vi "GE 5565PIORC.DMA.Scatter-Gather.Link Block Descriptors.vi"(8 "error in (no error)":errorcluster, 10 "Block Descriptors":T1[](array[typedef]) {"descriptor params"."data ptr (lower)" format="%.0x"; "descriptor params"."data ptr (upper)" format="%.0x"; "descriptor params"."data size" format="%.0x"; "descriptor params"."next descriptor ptr" format="%.0x"; "descriptor size" format="%08x"; "descriptor ptr (RFM)" format="%08x"; "descriptor ptr (VISA)" format="%08x"}, 11 "GE 5565PIORC in":refnum<class "GE 5565PIORC.lvclass">) -> (0 "error out":errorcluster, 2 "Linked Block Descriptors":T1[](array[typedef]) {"descriptor params"."data ptr (lower)" format="%.0x"; "descriptor params"."data ptr (upper)" format="%.0x"; "descriptor params"."data size" format="%.0x"; "descriptor params"."next descriptor ptr" format="%.0x"; "descriptor size" format="%08x"; "descriptor ptr (RFM)" format="%08x"; "descriptor ptr (VISA)" format="%08x"}, 3 "GE 5565PIORC out":refnum<class "GE 5565PIORC.lvclass">)   [LabVIEW 2020, in "GE 5565PIORC.lvclass"]
doc: "Modifies the pointers for each Block Descriptor in the <B>Block Descriptors</B> array to ensure that each element points to the location of the next descriptor in memory."
uses:
  GE 5565PIORC.lvclass
  Typedefs/GE 5565PIORC.Typedef.DMA Block Descriptor.ctl
  Typedefs/GE 5565PIORC.Typedef.DMA Block Descriptor Params.ctl
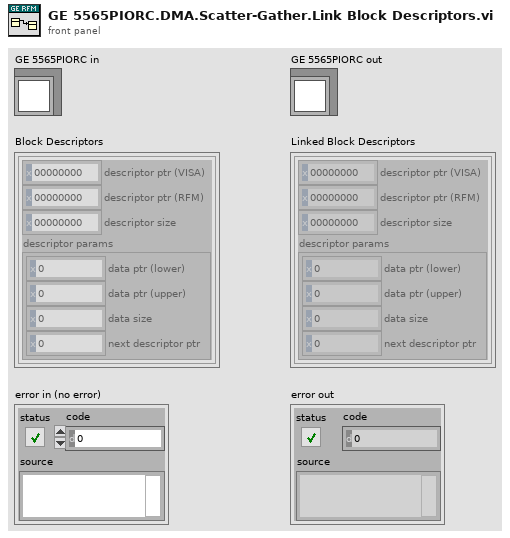
[diagram p1: front panel]
types:
  T1 = typedef "GE 5565PIORC.lvclass/GE 5565PIORC.Typedef.DMA Block Descriptor.ctl" = cluster{"descriptor ptr (VISA)":u32, "descriptor ptr (RFM)":u32, "descriptor size":u32, "descriptor params":T2}
  T2 = typedef "GE 5565PIORC.lvclass/GE 5565PIORC.Typedef.DMA Block Descriptor Params.ctl" = cluster{"data ptr (lower)":u32, "data ptr (upper)":u32, "data size":u32, "next descriptor ptr":u32}
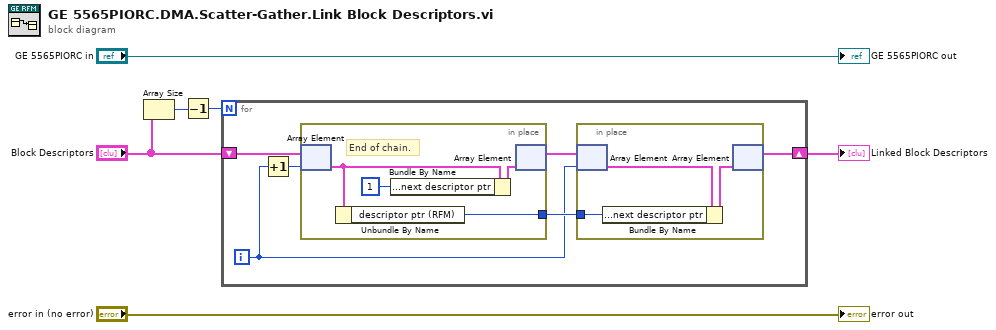
[diagram p0: block diagram]
diagram:
  n1 = Array Size(array="Block Descriptors") -> (size(s)=w5:i32)
  n2 = Decrement(x=w5) -> (x-1=w4:i32)
  n3 = for {
    N: w4 -> [_]
    shift-right: [w9] -> w2
    shift-left: "Block Descriptors" -> [w11]
    i -> [w7]
    n4 = Increment(x=w7) -> (x+1=w12:i32)
    n5 = in-place {
      in-place-border: [w13] -> w8
      # "End of chain."
      n6 = in-place-array #1(w11, w12) -> (w16:T1)
      n7 = Unbundle By Name(w16) -> ("descriptor ptr (RFM)"=w13:u32)
      n8 = Bundle By Name(cluster=w16, "descriptor params.next descriptor ptr"=u32 1 ("next descriptor ptr")) -> (w15:T1)
      n9 = in-place-array #1(w15) -> (w10:T1[])  [unwired: 1 out]
    }
    n10 = in-place {
      in-place-border: w8 -> [w17]
      n11 = in-place-array #2(w10, w7) -> (w19:T1)
      n12 = Bundle By Name(cluster=w19, "descriptor params.next descriptor ptr"=w17) -> (w18:T1)
      n13 = in-place-array #2(w18) -> (w9:T1[])  [unwired: 1 out]
    }
  }
  "Linked Block Descriptors" <- w2
  "error out" <- "error in (no error)"
  "GE 5565PIORC out" <- "GE 5565PIORC in"
